vi "session_set_instrument_options.vi"(8 "error in":errorcluster, 10 "Options string":string, 11 "VISA resource name":refnum<visa-resource-name>) -> (0 "error out":errorcluster, 3 "VISA resource name out":refnum<visa-resource-name>)   [LabVIEW 2014, in "rszvl_rsidr_core.lvlib"]
uses:
  rszvl_rsidr_core.lvlib
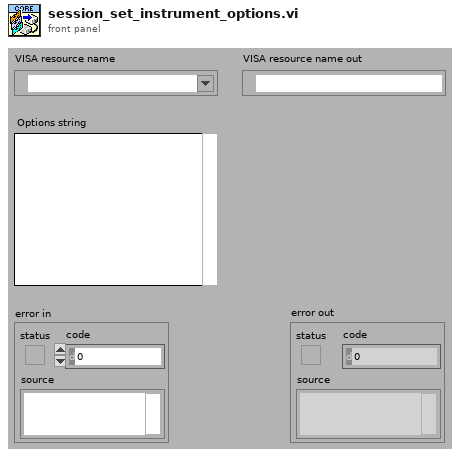
[diagram p1: front panel]
types:
  T1 = typedef "rszvl_rsidr_core.lvlib/type_Session_Data.ctl" = cluster{"Instr type":string, "Instr type for err. msg.":string, "Installed Options":string[], "OPC Timeout":i32, "Query Instrument Status":bool, "Check Range":bool, "Check Options":bool, "Add LF to Write":bool, "Simulate":bool, "Logging":bool, "Logging params":variant, "Interface Type":enum16{"Unknown", "GPIB", "VXI", "GPIB_VXI", "ASRL", "PXI", "TCPIP", "USB", "SOCKET"}, "Fast Sweep":i32, "AdditionalFlags":i32, "WaitBeforeWrite":i32, "WaitBeforeRead":i32, "BinDataChunkSize":i64}
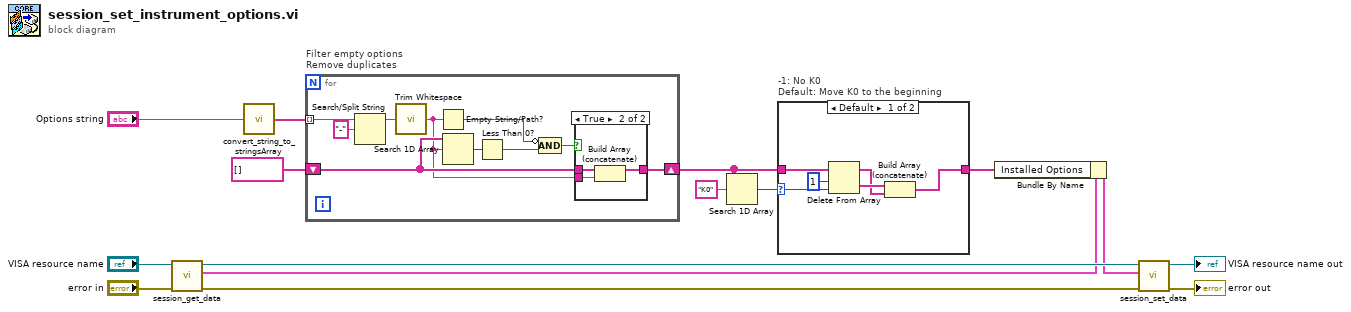
[diagram p0: block diagram]
diagram:
  n1 = call "session_get_data.vi"("error in"="error in", "VISA resource name"="VISA resource name") -> ("error out"=w11:errorcluster, "Session User Data out"=w6:T1, "VISA resource name out"=w10:refnum<visa-resource-name>)  [unwired: 7 in]
  n2 = call "convert_string_to_stringsArray.vi"("String in"="Options string") -> ("string array out"=w14:string[])  [unwired: 3 in, 1 out]
  n3 = for "Filter empty options\nRemove duplicates" {
    tunnel: w14 -> [w16] mode=indexing
    shift-right: [w25] -> w2
    shift-left: string[] [] -> [w22]
    n4 = Search/Split String(string=w16, search string/char (-)="-" ("regular expression")) -> (substring before match=w23:string)  [unwired: 1 in, 2 out]
    n5 = call "Trim Whitespace.vi"("string"=w23) -> ("trimmed string"=w21:string)  [unwired: 1 in]
    n6 = Empty String/Path?(string/path=w21) -> (empty?=w17:bool)
    n7 = Search 1D Array(1D array=w22, element=w21) -> (index of element=w19:i32)  [unwired: 1 in]
    n8 = Less Than 0?(x=w19) -> (x < 0?=w20:bool)
    n9 = Compound Arithmetic op=AND(invert w17, w20) -> (w18:bool)
    n10 = case shown="True" w18 {
      tunnel: [w26 w27] -> w25
      tunnel: w22 -> [w26 w29]
      tunnel: w21 -> [_ w28]
      frame False {
      }
      frame True {
        n11 = Build Array (concatenate)(w29, w28) -> (w27:string[])
      }
    }
  }
  n12 = Search 1D Array(1D array=w2, element="K0") -> (index of element=w3:i32)  [unwired: 1 in]
  n13 = case "-1: No K0\nDefault: Move K0 to the beginning" shown="Default" w3 {
    selector: w3 -> [w34 _]
    tunnel: w2 -> [w35 w36]
    tunnel: [w32 w36] -> w1
    frame Default {
      n14 = Delete From Array(array=w35, length=1, index=w34) -> (deleted portion=w31:string[], array with subset deleted=w30:string[])
      n15 = Build Array (concatenate)(w31, w30) -> (w32:string[])
    }
    frame -1 {
    }
  }
  n16 = Bundle By Name(cluster=w6, "Installed Options"=w1) -> (w7:T1)
  n17 = call "session_set_data.vi"("error in"=w11, "Session User Data in"=w7, "VISA resource name"=w10) -> ("error out"=→"error out":errorcluster, "VISA resource name out"=→"VISA resource name out":refnum<visa-resource-name>)  [unwired: 7 in]
